vi "SIAM_type.vi"() -> ()   [LabVIEW 2011]
panel:
  out "error out":errorcluster
  out "net address":u32
  in  "name":string
  out "connection ID out":refnum<k5>
  in  "connection ID":refnum<k5>
  in  "#Entries":i32
  in  "Script":T1(array[cluster])=[{"command"=4027514895, "Delay 10µs"=0, "P0"=16777215, "P1"=0, "P2"=0, "P3"=0, "P4"=0, "P5-ticket"=0}, {"command"=4027514895, "Delay 10µs"=0, "P0"=100, "P1"=0, "P2"=0, "P3"=0, "P4"=0, "P5-ticket"=0}, {"command"=4027514895, "Delay 10µs"=0, "P0"=5, "P1"=120, "P2"=0, "P3"=0, "P4"=0, "P5-ticket"=0}] {"command" format="%x" items=["read_x-Motor_status_ticket"=17305600, "init_x-Motor"=17760263, "read_x-Motor_absolute_ticket"=16781312, "move_x-Motor_absolute"=16777217, "move_x-Motor_relative"=16842753, "read y-Motor status, ticket"=18354176, "init y-Motor"=18808839, "read y-Motor absolute, ticket"=17829888, "move y-Motor absolute"=17825793, "move y-Motor relative"=17891329, "read z-Motor status, ticket"=19402752, "init z-Motor"=19857415, "stop z-Motor"=19857423, "start z-Motor"=19857422, "read z-Motor absolute, ticket"=18878464, "move z-Motor absolute"=18874369, "move z-Motor relative"=18939905, "end_no_ticket"=4027514895, "end_ticket"=4027518991, "IO-read_bank0"=218107904, "IO-write_bank0"=218103809, "IO-read_bank1"=219156480, "IO-write_bank1"=219152385, "IO-delay_bank0"=218365953, "IO-delay_bank0_fromVar"=218365955, "read_cam_clock"=3289124864, "set_cam_deadtime"=3288989697, "set_cam_10uscycles"=3289055233, "calc_cam"=3289317386, "store_cam_Var"=3289251842, "math_substractFromVariable"=4060086278, "readVar"=4060090368, "writeVar"=4060086273, "copyVar"=4060086276, "decrement_branchRel_if_greater"=4043374945, "decrement_branchRel_if_greaterequal"=4043375201, "writeTMSI"=100663297, "writeTMSI_fromVar"=100663299]}
  in  "allow movement from end":i32
  in  "allowed start movement":i32
  in  "max. Estimate/Deterministic":bool
  in  "Duration Ticks":i32
  in  "Fixed Base Adress (<>0)":dbl
  # "run command\nwrite protocol, read protocol?\nrun protokol\nread status (running.., ticket available..errorcodes..) - braucht zwingend anschluss zum READ!\n\nread ticketvalue\nread ticketarray\ncreate/clear ticket\n\ntimersynchronizartion?\n\nopen close? openID. freeID"
  # "need a background service with queue? writ no, read???\nnur wenn ich schnell auf antworten reagieren müsste IRQ\nein warten auf.. geht mit klassiaschem sub-vi nicht (non-reentrant, non-blocking)"
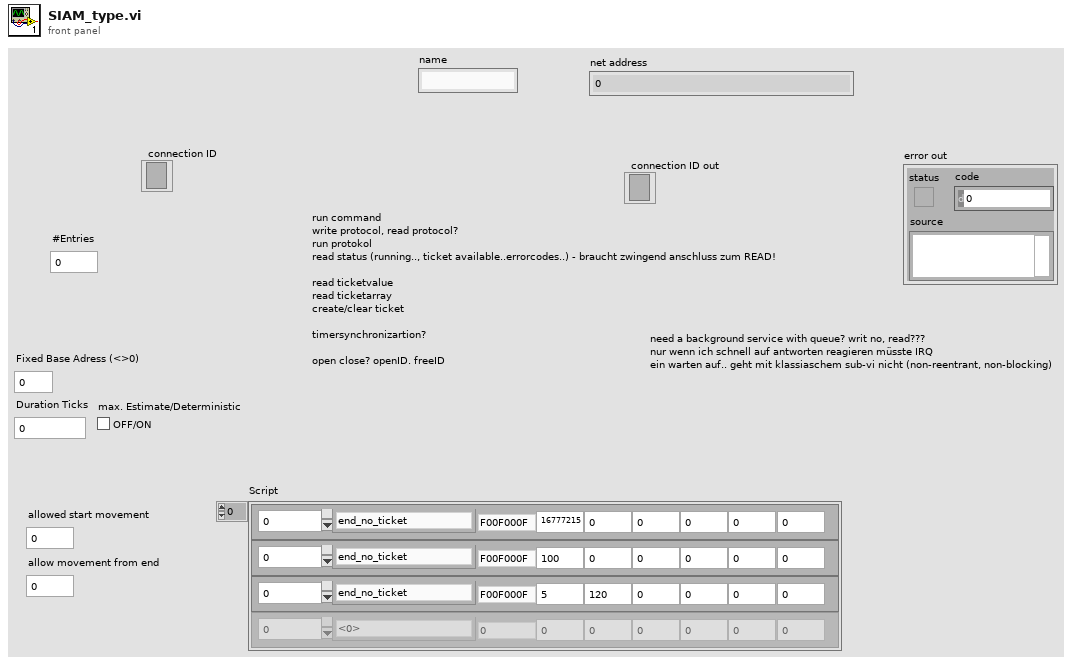
[diagram p1: front panel]
types:
  T1 = cluster{"command":u32, "Delay 10µs":u32, "P0":i32, "P1":i32, "P2":i32, "P3":i32, "P4":i32, "P5-ticket":i32}[]
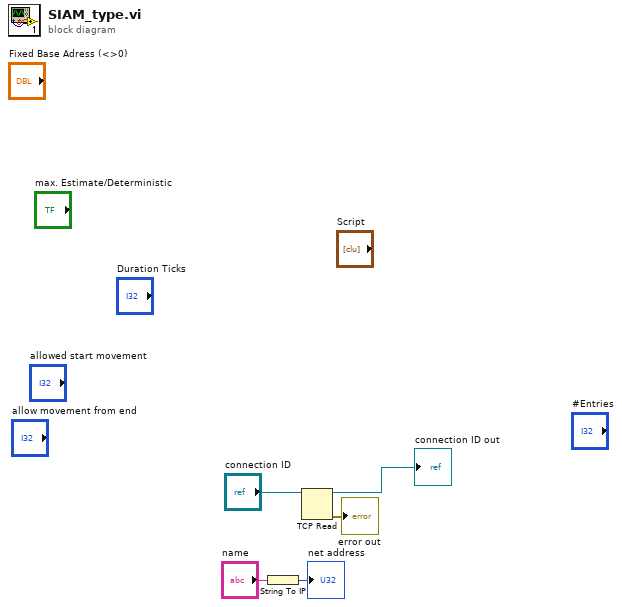
[diagram p0: block diagram]
diagram:
  n1 = String To IP(1:"name") -> (0:→"net address":u32)
  n2 = TCP Read(connection ID="connection ID") -> (connection ID out=→"connection ID out":refnum<k5>, error out=→"error out":errorcluster)  [unwired: 4 in, 1 out]
